vi "Store images.vi"(6 "ms Capture Rate":u32=100, 8 "# Total images IN":i32, 9 "# new images to capture":i32, 10 "Store # Images?":bool, 11 "Image":T1) -> (0 "Total images OUT":i32, 3 "Image Out":T1)   [LabVIEW 2018]
uses:
  <vilib>/vision/Image Controls.llb/IMAQ Image.ctl
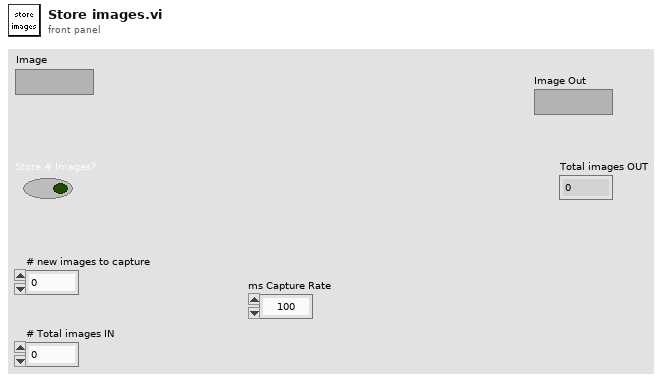
[diagram p1: front panel]
types:
  T1 = typedef "IMAQ Image.ctl" = refnum<image>
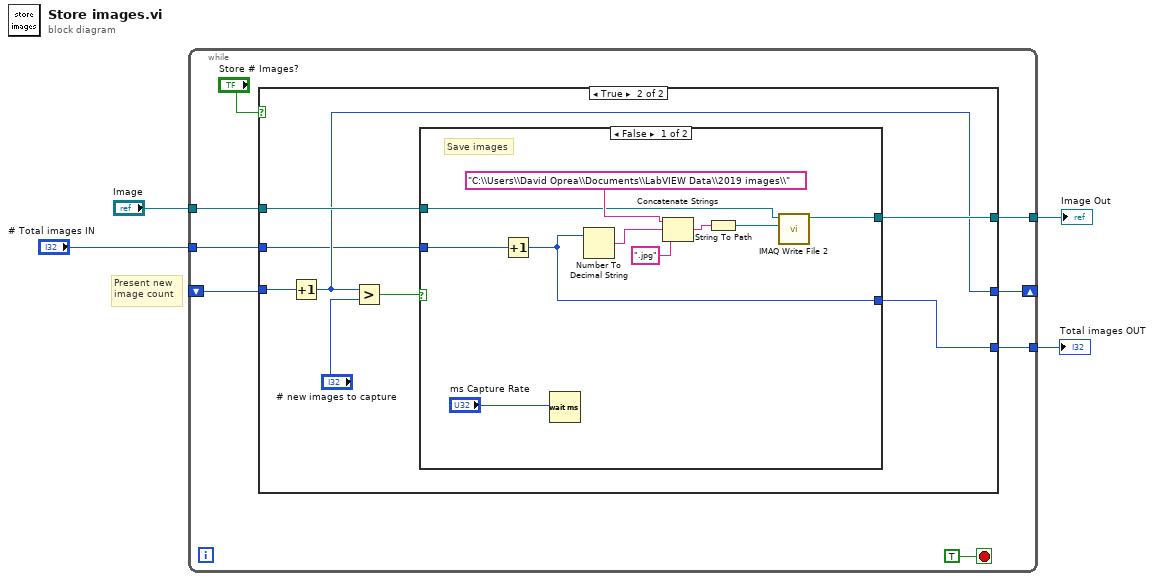
[diagram p0: block diagram]
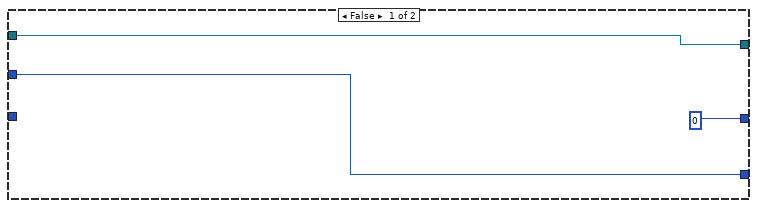
[diagram p2: hidden frame]
diagram:
  # "Present new\nimage count"
  n1 = while {
    tunnel: "Image" -> [w11]
    tunnel: [w9] -> w3
    shift-right: [w8] -> _
    shift-left: _ -> [w7]
    tunnel: [w6] -> w2
    tunnel: "# Total images IN" -> [w5]
    stop <- TRUE stop-if-true
    n2 = case shown="True" "Store # Images?" {
      tunnel: w7 -> [_ w19]
      tunnel: w11 -> [w15 w23]
      tunnel: [w15 w22] -> w9
      tunnel: [0 w18] -> w8
      tunnel: [w13 w17] -> w6
      tunnel: w5 -> [w13 w16]
      frame False {
      }
      frame True {
        n3 = Increment(x=w19) -> (x+1=w18:i32)
        n4 = Greater?(x=w18, y="# new images to capture") -> (0:w21:bool)
        n5 = case shown="False" w21 {
          tunnel: w23 -> [w28 w35]
          tunnel: [w27 w35] -> w22
          tunnel: [w25 w34] -> w17
          tunnel: w16 -> [w24 w34]
          frame False {
            # "Save images"
            n6 = Increment(x=w24) -> (x+1=w25:i32)
            n7 = Wait (ms)(milliseconds to wait="ms Capture Rate") -> ()  [unwired: 1 out]
            n8 = Number To Decimal String(number=w25) -> (decimal integer string=w33:string)  [unwired: 1 in]
            n9 = Concatenate Strings("C:\\Users\\David Oprea\\Documents\\LabVIEW Data\\2019 images\\", w33, ".jpg") -> (w31:string)
            n10 = String To Path(string=w31) -> (path=w29:path)
            n11 = call-poly "IMAQ Write File 2"("File Path"=w29, "Image"=w28) -> ("Image Out (duplicate)"=w27:T1)  [unwired: 8 in, 1 out]
          }
          frame True {
            # "Do not save images"
          }
        }
      }
    }
  }
  "Image Out" <- w3
  "Total images OUT" <- w2
